vi "n jump rel 3d.vi"(7 "dz":i16, 8 "error in (no error)":errorcluster, 9 "dy":i16, 10 "dx":i16, 11 "n":u16) -> (0 "error out":errorcluster)   [LabVIEW 2015, in "SCANalone4x64.lvlib"]
doc: "__declspec(dllimport) void __stdcall n_jump_rel_3d(unsigned short n, short dx, short dy, short dz);"
uses:
  <userlib>/SCANalone4x64/SCANalone4x64.lvlib
  <userlib>/SCANalone4x64/SCANalone4x64.dll
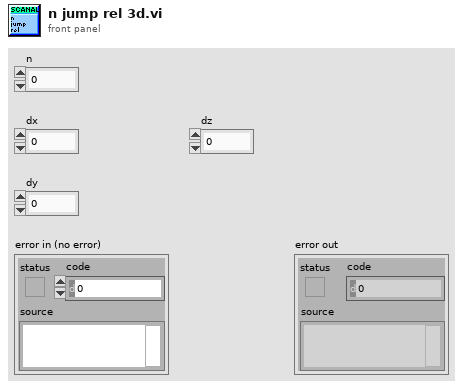
[diagram p1: front panel]
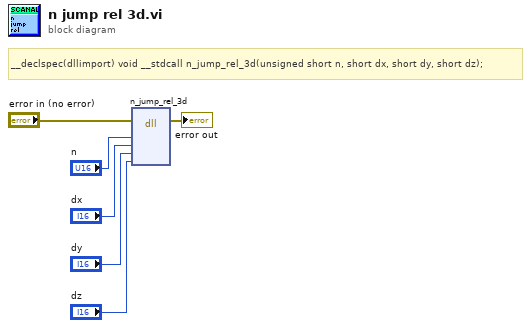
[diagram p0: block diagram]
diagram:
  # "__declspec(dllimport) void __stdcall n_jump_rel_3d(unsigned short n, short dx, short dy, short dz);"
  n1 = dll-call lib="C:/Program Files/National Instruments/LabVIEW 2015/user.lib/SCANalone4x64/SCANalone4x64.*" fn="n_jump_rel_3d"(error in="error in (no error)", "n"="n", "dx"="dx", "dy"="dy", "dz"="dz") -> (error out=→"error out":errorcluster)  [unwired: 7 in, 1 out]
